vi "ble_rsp_gap_end_procedure.vi"(8 "error in (no error)":errorcluster, 11 "COM Bluegiga in":refnum<visa-resource-name>) -> (0 "error out":errorcluster, 1 "success?":bool, 2 "full message package":u8[](array[numeric]), 3 "COM Bluegiga out":refnum<visa-resource-name>)   [LabVIEW 2015]
uses:
  type_def/message_class.ctl
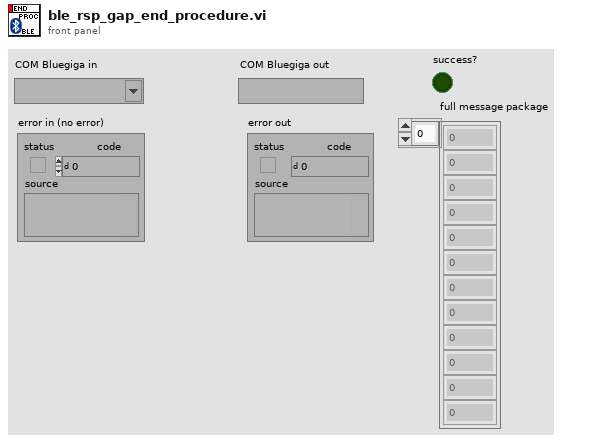
[diagram p1: front panel]
types:
  T1 = typedef "message_class.ctl" = u8
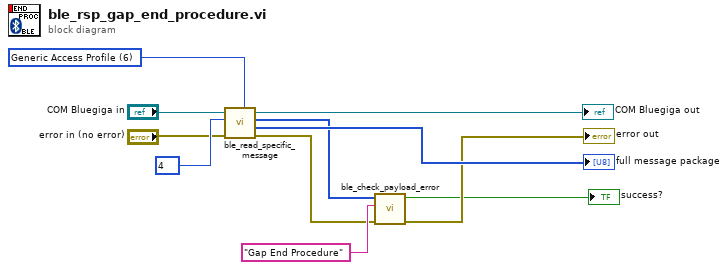
[diagram p0: block diagram]
diagram:
  w9 = T1 6 items=["System", "Persistent Store", "Attribute database", "Connection", "Attribute client", "Security Manager", "Generic Access Profile", "Hardware"] ("Command Class (System)")
  n1 = call "ble_read_specific_message.vi"("Command Class (System)"=w9, "error in (no error)"="error in (no error)", "Message ID (0x00)"=u8 4, "COM Bluegiga in"="COM Bluegiga in") -> ("error out"=w1:errorcluster, "full message package"=→"full message package":u8[], "specific payload"=w4:u8[], "COM Bluegiga out"=→"COM Bluegiga out":refnum<visa-resource-name>)  [unwired: 3 in, 1 out]
  n2 = call "ble_check_payload_error.vi"("error in (no error)"=w1, "error source"="Gap End Procedure", "payload"=w4) -> ("error out"=→"error out":errorcluster, "success?"=→"success?":bool)  [unwired: 7 in]
